vi "Sort Alarms.vi"(11 "alarms":T2(array[cluster]) {"value" format="%.2f"; "setpoint" format="%.2f"; "clear time" format="%<%X\n%x>T"; "ack time" format="%<%X\n%x>T"; "set time" format="%<%X\n%x>T"}) -> (3 "alarms out":T2(array[cluster]) {"value" format="%.2f"; "setpoint" format="%.2f"; "clear time" format="%<%X\n%x>T"; "ack time" format="%<%X\n%x>T"; "set time" format="%<%X\n%x>T"})   [LabVIEW 2021, in "Dynamic Shared Variables.lvlib"]
doc: "Sort alarms per Delta V alarm ranking."
uses:
  Dynamic Shared Variables.lvlib
panel:
  out "Array":T1(array[cluster])
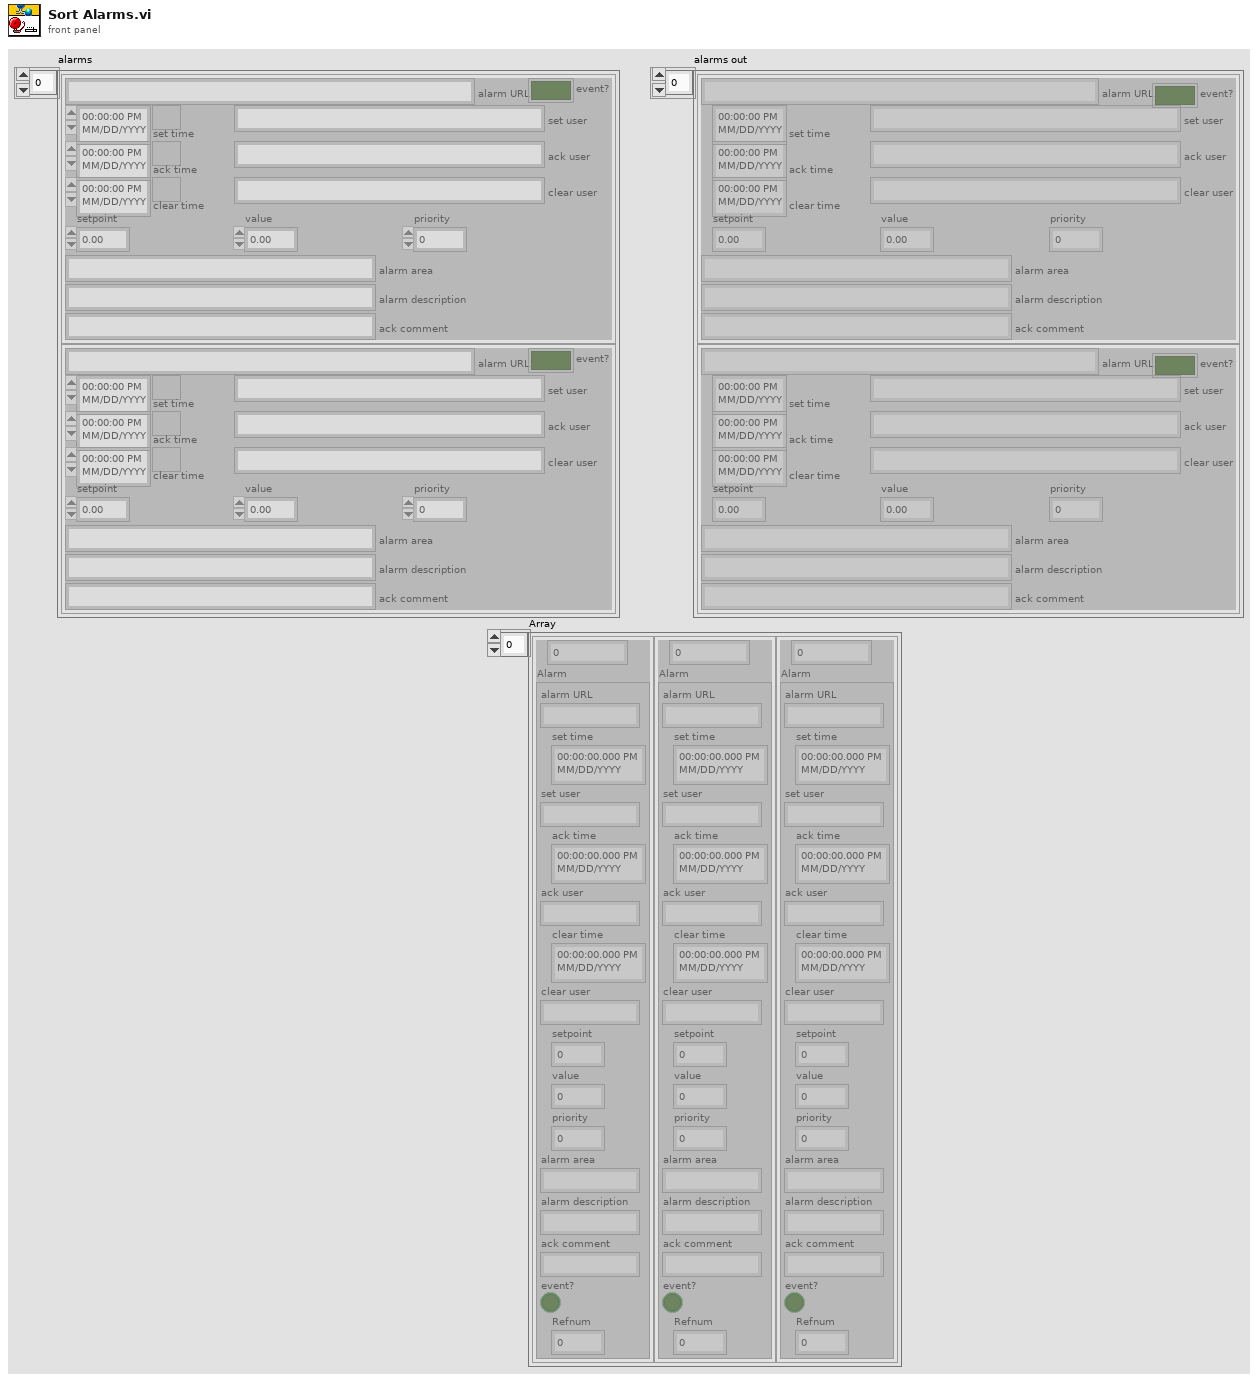
[diagram p1: front panel]
types:
  T1 = cluster{ext, "Alarm":cluster{"alarm URL":string, "set time":timestamp, "set user":string, "ack time":timestamp, "ack user":string, "clear time":timestamp, "clear user":string, "setpoint":dbl, "value":dbl, "priority":u32, "alarm area":string, "alarm description":string, "ack comment":string, "event?":bool, "Refnum":u64}}[]
  T2 = cluster{"alarm URL":string, "set time":timestamp, "set user":string, "ack time":timestamp, "ack user":string, "clear time":timestamp, "clear user":string, "setpoint":dbl, "value":dbl, "priority":u32, "alarm area":string, "alarm description":string, "ack comment":string, "event?":bool, "Refnum":u64}[]
  T3 = cluster{ext, "Alarm":cluster{"alarm URL":string, "set time":timestamp, "set user":string, "ack time":timestamp, "ack user":string, "clear time":timestamp, "clear user":string, "setpoint":dbl, "value":dbl, "priority":u32, "alarm area":string, "alarm description":string, "ack comment":string, "event?":bool, "Refnum":u64}}
  T4 = cluster{"alarm URL":string, "set time":timestamp, "set user":string, "ack time":timestamp, "ack user":string, "clear time":timestamp, "clear user":string, "setpoint":dbl, "value":dbl, "priority":u32, "alarm area":string, "alarm description":string, "ack comment":string, "event?":bool, "Refnum":u64}
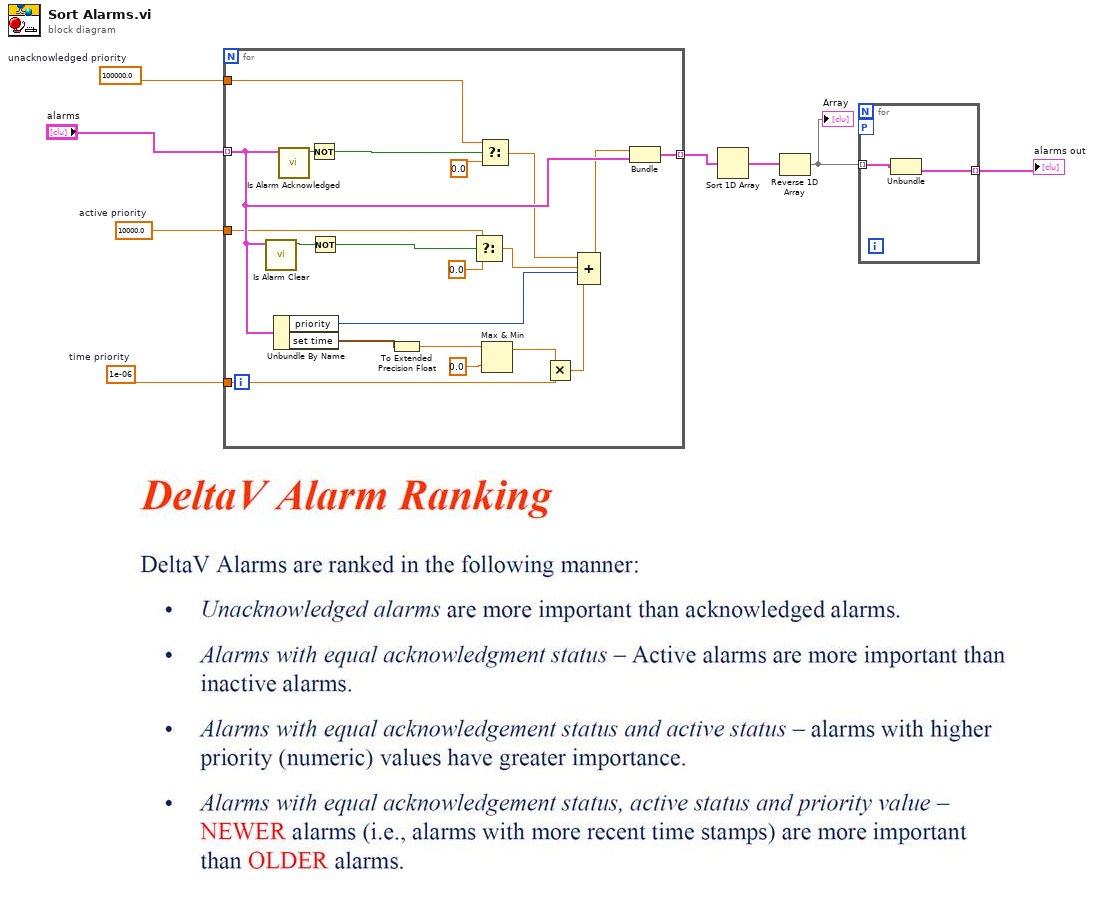
[diagram p0: block diagram]
diagram:
  w5 = 1e-06  # time priority
  w6 = 10000.0  # active priority
  w7 = 100000.0  # unacknowledged priority
  n1 = for {
    tunnel: "alarms" -> [w27] mode=indexing
    tunnel: w7 -> [w22]
    tunnel: w6 -> [w26]
    tunnel: w5 -> [w14]
    tunnel: [w10] -> w4 mode=indexing
    n2 = call "Is Alarm Clear.vi"("Alarm"=w27) -> ("Cleared?"=w25:bool)  [unwired: 10 in]
    n3 = Unbundle By Name(w27) -> ("priority"=w18:u32, "set time"=w16:timestamp)
    n4 = call "Is Alarm Acknowledged.vi"("Alarm"=w27) -> ("Acknowledged?"=w28:bool)  [unwired: 8 in, 2 out]
    n5 = Not(x=w28) -> (.not. x?=w24:bool)
    n6 = Not(x=w25) -> (.not. x?=w9:bool)
    n7 = To Extended Precision Float(1:w16) -> (0:w15:ext)
    n8 = Select(t=w26, s=w9, f=0.0 ("t")) -> (s? t:f=w19:dbl)
    n9 = Select(t=w22, s=w24, f=0.0 ("t")) -> (s? t:f=w20:dbl)
    n10 = Max & Min(x=w15, y=0.0 ("t")) -> (max(x,y)=w13:ext)  [unwired: 1 out]
    n11 = Multiply(x=w13, y=w14) -> (x*y=w12:ext)
    n12 = Compound Arithmetic op=ADD(w20, w19, w18, w12) -> (w11:ext)
    n13 = Bundle(w11, "Alarm"=w27) -> (w10:T3)  [unwired: 1 in]
  }
  n14 = Sort 1D Array(array=w4) -> (sorted array=w3:T1)
  n15 = Reverse 1D Array(array=w3) -> (reversed array=w1:T1)
  "Array" <- w1
  n16 = for {
    tunnel: w1 -> [w30] mode=indexing
    tunnel: [w29] -> w2 mode=indexing
    workers-P: _ -> [_]
    n17 = Unbundle(w30) -> ("Alarm"=w29:T4)  [unwired: 1 out]
  }
  "alarms out" <- w2
